vi "ToggleMode.vi"(8 "error in (no error)":errorcluster, 10 "Mode":T1, 11 "Pod Drive in":refnum<class "Pod Drive.lvclass">) -> (0 "error out":errorcluster, 3 "Pod Drive out":refnum<class "Pod Drive.lvclass">)   [LabVIEW 2018, in "Drive.lvlib" / "Pod Drive.lvclass"]
doc: "Configures the talons based on weather your running closed loop velocity mode or motion magic"
uses:
  Pod Drive.lvclass
  Controls/Mode.ctl
  Pod Drive.lvclass/Pod Drive.ctl
  Drive.lvclass
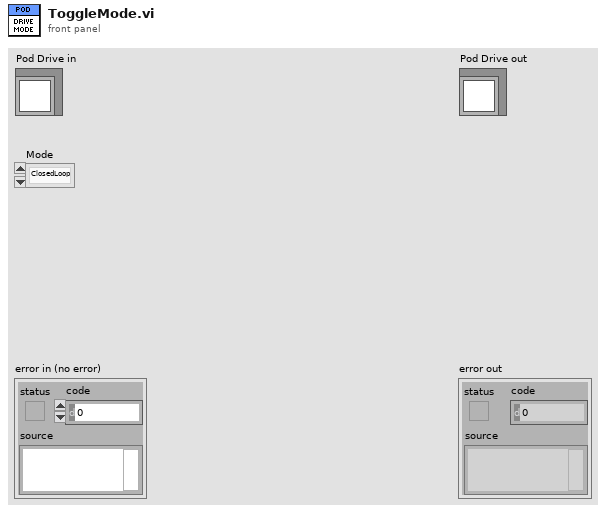
[diagram p1: front panel]
types:
  T1 = typedef "Drive.lvlib/Pod Drive.lvclass/Mode.ctl" = enum16{"ClosedLoop", "MotionMagic"}
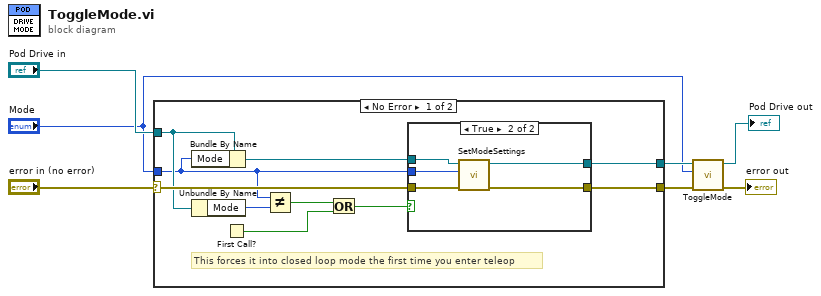
[diagram p0: block diagram]
diagram:
  n1 = case shown="No Error" "error in (no error)" {
    selector: "error in (no error)" -> [w17 w26]
    tunnel: [w16 w26] -> w4
    tunnel: [w10 w25] -> w5
    tunnel: "Pod Drive in" -> [w14 w25]
    tunnel: "Mode" -> [w13 _]
    frame No Error {
      # "This forces it into closed loop mode the first time you enter teleop"
      n2 = Bundle By Name(cluster=w14, "Mode"=w13) -> (w11:refnum<class "Pod Drive.lvclass">)
      n3 = Unbundle By Name(w14) -> ("Mode"=w12:T1)
      n4 = First Call?() -> (First Call?: T/F=w8:bool)
      n5 = Not Equal?(x=w13, y=w12) -> (x != y?=w15:bool)
      n6 = Or(x=w15, y=w8) -> (x .or. y?=w9:bool)
      n7 = case shown="True" w9 {
        tunnel: w17 -> [w19 w24]
        tunnel: [w19 w23] -> w16
        tunnel: w13 -> [_ w22]
        tunnel: w11 -> [w18 w21]
        tunnel: [w18 w20] -> w10
        frame False {
        }
        frame True {
          n8 = call "SetModeSettings.vi"("error in (no error)"=w24, "Mode"=w22, "Drive.lvlib:Pod Drive.lvclass"=w21) -> ("error out"=w23:errorcluster, 3:w20:refnum<class "Pod Drive.lvclass">)  [unwired: 7 in]
        }
      }
    }
    frame Error {
    }
  }
  n9 = call-parent "ToggleMode.vi"("error in (no error)"=w4, "Mode"="Mode", "Drive in"=w5) -> ("error out"=→"error out":errorcluster, "Drive out"=→"Pod Drive out":refnum<class "Pod Drive.lvclass">)  [unwired: 7 in]
